vi "Send Image.vi"(7 "image filepath":path, 8 "error in (no error)":errorcluster, 9 "slack channel":string, 10 "slack API token":string) -> (0 "error out":errorcluster, 1 "slack channel dup":string, 2 "slack API token dup":string)   [LabVIEW 2018, in "Slack API.lvlib"]
uses:
  Slack API.lvlib
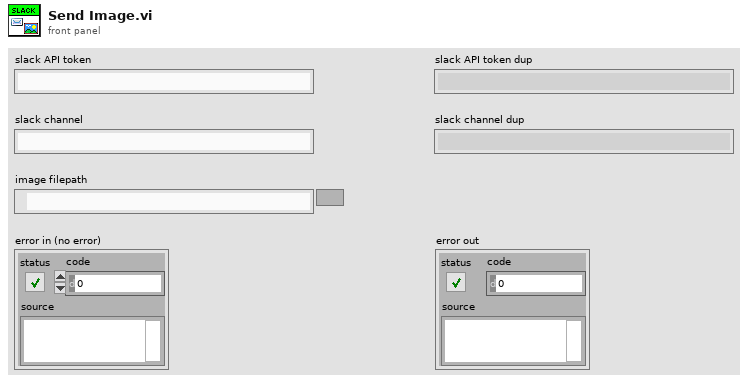
[diagram p1: front panel]
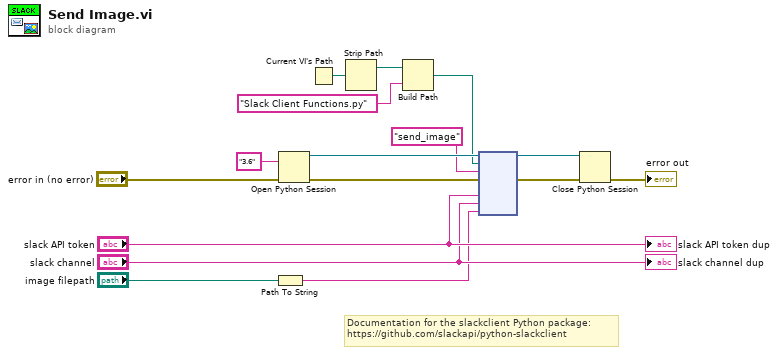
[diagram p0: block diagram]
diagram:
  # "Documentation for the slackclient Python package:\nhttps://github.com/slackapi/python-slackclient"
  n1 = Path To String(path="image filepath") -> (string=w1:string)
  n2 = Open Python Session(python version="3.6" ("Python version"), 3:"error in (no error)") -> (session out=w15:refnum<k35>, error out=w13:errorcluster)  [unwired: 1 in]
  n3 = Current VI's Path() -> (path=w9:path)
  n4 = Strip Path(path=w9) -> (stripped path=w8:path)  [unwired: 1 out]
  n5 = Build Path(base path=w8, name or relative path="Slack Client Functions.py") -> (appended path=w7:path)
  n6 = node(w15, w7, "send_image" ("function name"), w13, "slack API token", "slack channel", w1) -> (w10:refnum<k35>, w11:errorcluster)  [unwired: 5 in, 2 out]
  n7 = Close Python Session(session in=w10, error in=w11) -> (11:→"error out":errorcluster)
  "slack API token dup" <- "slack API token"
  "slack channel dup" <- "slack channel"
